vi "4ship.vi"(0 "Array":u16[][](array[ring])) -> (2 "Array 2":u16[][](array[ring]))   [LabVIEW 2014]
panel:
  in  "Array 8":u16[][](array[ring])=[[1, 1, 1, 1]]
  in  "Array 9":u16[][](array[ring])=[[1], [1], [1], [1]]
  out "Boolean":bool
  in  "Raw":i32=1
  in  "Column":i32=1
  in  "?":bool
  in  "?":enum16{"horizon", "vertical"}(ring)
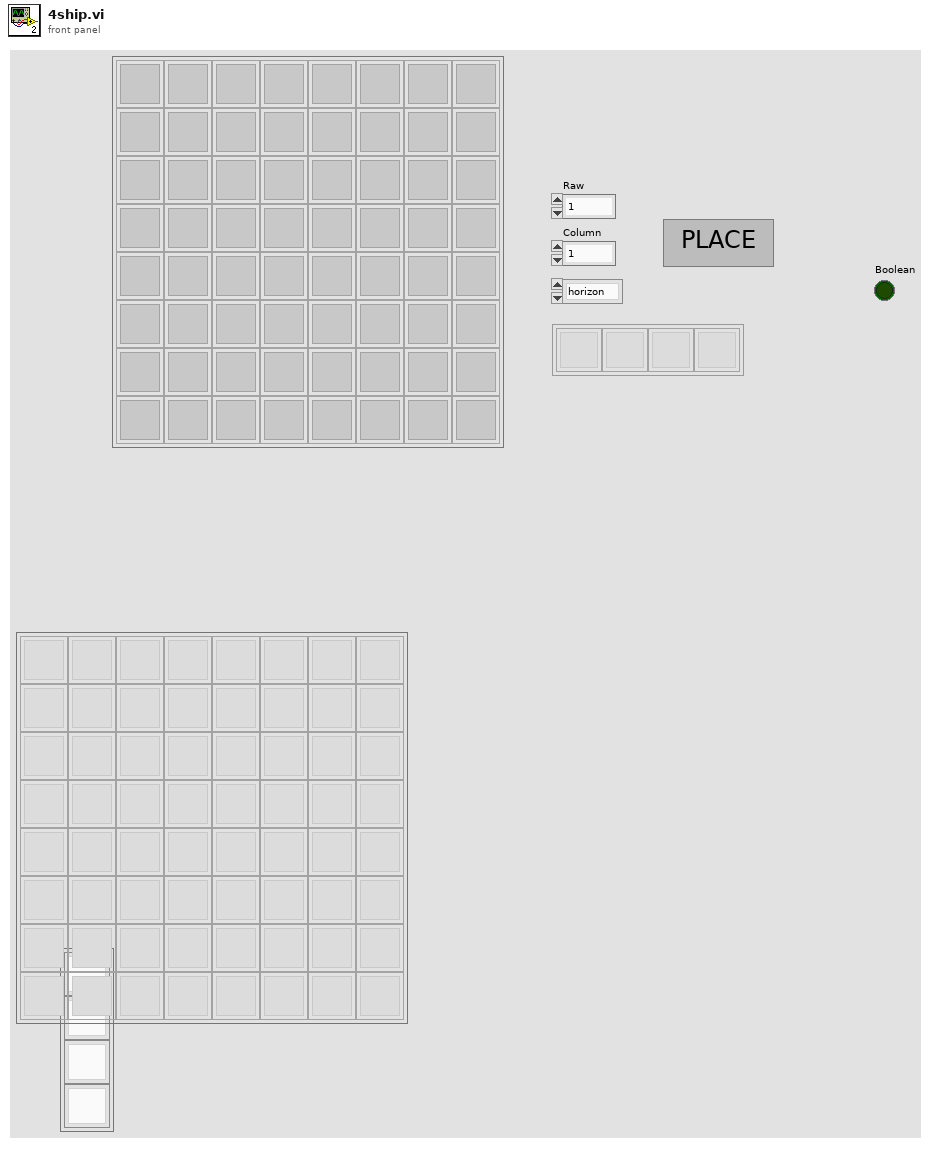
[diagram p1: front panel]
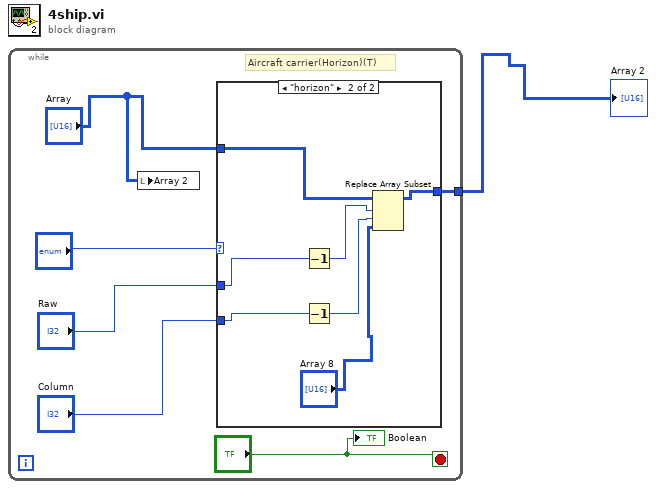
[diagram p0: block diagram]
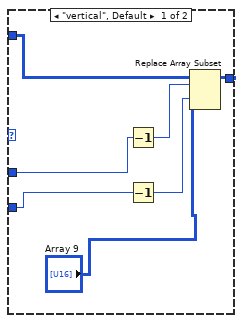
[diagram p2: hidden frame]
diagram:
  n1 = while {
    tunnel: [w7] -> w1
    stop <- "?" stop-if-true
    # "Aircraft carrier(Horizon)(T)"
    n2 = local write "Array 2"("Array") -> ()
    n3 = case shown="\"horizon\"" "?" {
      tunnel: [w12 w19] -> w7
      tunnel: "Raw" -> [w11 w18]
      tunnel: "Column" -> [w10 w17]
      tunnel: "Array" -> [w9 w16]
      frame "vertical", Default {
        n4 = Decrement(x=w11) -> (x-1=w14:i32)
        n5 = Decrement(x=w10) -> (x-1=w13:i32)
        n6 = Replace Array Subset(array=w9, new element="Array 9", index (row)=w14, index (col)=w13) -> (w12:u16[][])
      }
      frame "horizon" {
        n7 = Decrement(x=w18) -> (x-1=w21:i32)
        n8 = Decrement(x=w17) -> (x-1=w20:i32)
        n9 = Replace Array Subset(array=w16, new element="Array 8", index (row)=w21, index (col)=w20) -> (w19:u16[][])
      }
    }
    "Boolean" <- "?"
  }
  "Array 2" <- w1
